vi "Simple Event Driven Example.vi"() -> ()   [LabVIEW 2013]
uses:
  lightfield-automation-labview/LightField Automation.lvclass
panel:
  in  "Load":bool
  in  "Experiment Name":string
  in  "Preview":bool
  in  "Acquire":bool
  in  "Exposure Time (s)":dbl format="%_3p"
  out "Intensity Graph":dbl[][](graph)
  in  "Close Program":bool
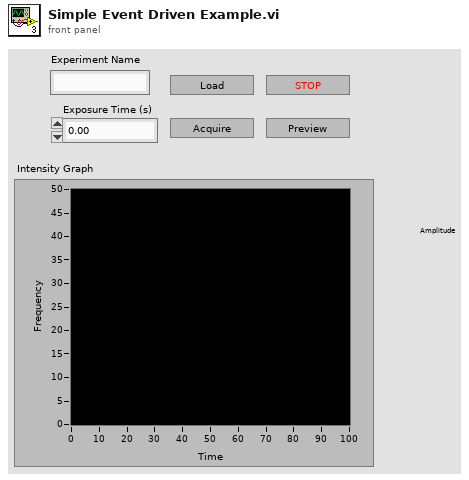
[diagram p1: front panel]
types:
  T1 = cluster{"Image":dbl[][][], "Frame Size":cluster{"F":i32, "Y":i32, "X":i32}}[]
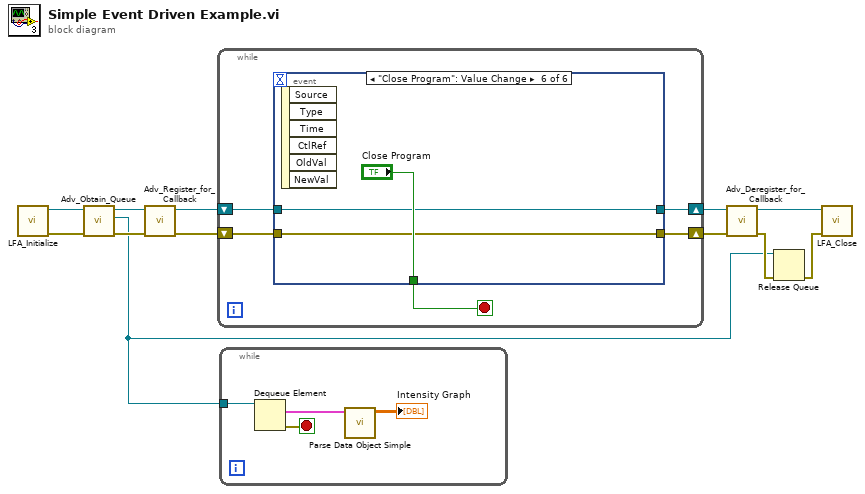
[diagram p0: block diagram]
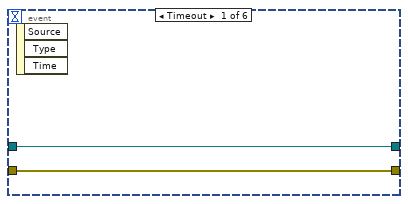
[diagram p2: hidden frame]
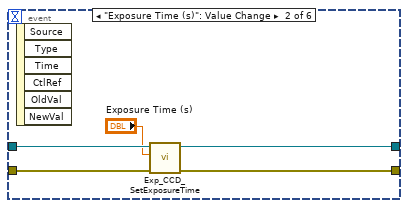
[diagram p3: hidden frame]
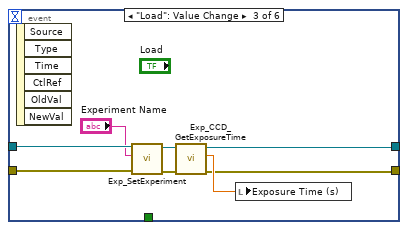
[diagram p4: hidden frame]
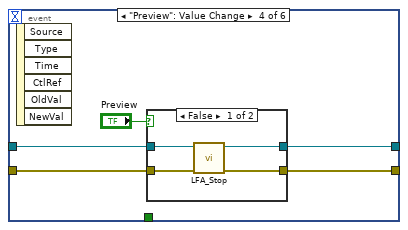
[diagram p5: hidden frame]
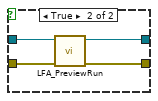
[diagram p6: hidden frame]
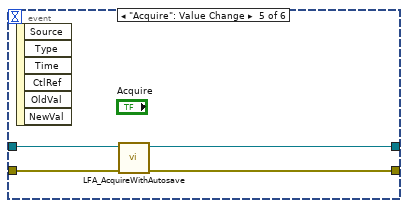
[diagram p7: hidden frame]
diagram:
  n1 = call "LFA_Initialize.vi"() -> ("error out"=w11:errorcluster, "LightField Automation out"=w12:refnum<class "LightField Automation.lvclass">)  [unwired: 10 in]
  n2 = call "Adv_Obtain_Queue.vi"("error in (no error)"=w11, "LightField Automation in"=w12) -> ("error out"=w9:errorcluster, "Queue Reference"=w1:refnum<queue>, "LightField Automation out"=w10:refnum<class "LightField Automation.lvclass">)  [unwired: 7 in]
  n3 = call "Adv_Register_for_Callback.vi"("error in (no error)"=w9, "LightField Automation in"=w10) -> ("error out"=w8:errorcluster, "LightField Automation out"=w7:refnum<class "LightField Automation.lvclass">)  [unwired: 8 in]
  n4 = while {
    shift-right: [w14] -> w6
    shift-left: w8 -> [w13]
    shift-right: [w15] -> w5
    shift-left: w7 -> [w16]
    stop <- w17 stop-if-true
    n5 = event shown="[5] \"Close Program\": Value Change" {
      selector: _ -> [_ _ _ _ _ _]
      dyn-events: _ -> [_ _ _ _ _ _]
      timeout: _ -> [_ _ _ _ _ _]
      tunnel: [_ _ _ _ _ "Close Program"] -> w17
      tunnel: w16 -> [w19 w24 w32 w34 w49 w51]
      tunnel: [w19 w21 w25 w35 w47 w51] -> w15
      tunnel: [w18 w22 w26 w36 w46 w50] -> w14
      tunnel: w13 -> [w18 w23 w31 w33 w48 w50]
      event Timeout {
        n6 = event-data() -> ()  [unwired: 1 in, 3 out]
      }
      event "Exposure Time (s)": Value Change {
        n7 = event-data() -> ()  [unwired: 1 in, 6 out]
        n8 = call "Exp_CCD_SetExposureTime.vi"("error in (no error)"=w23, "Exposure Time (s)"="Exposure Time (s)", "LightField Automation in"=w24) -> ("error out"=w22:errorcluster, "LightField Automation out"=w21:refnum<class "LightField Automation.lvclass">)  [unwired: 7 in]
      }
      event "Load": Value Change {
        n9 = event-data() -> ()  [unwired: 1 in, 6 out]
        n10 = call "Exp_SetExperiment.vi"("error in (no error)"=w31, "ExperimentName"="Experiment Name", "LightField Automation in"=w32) -> ("error out"=w29:errorcluster, "LightField Automation out"=w28:refnum<class "LightField Automation.lvclass">)  [unwired: 7 in]
        n11 = call "Exp_CCD_GetExposureTime.vi"("error in (no error)"=w29, "LightField Automation in"=w28) -> ("error out"=w26:errorcluster, "Exposure Time (s)"=w27:dbl, "LightField Automation out"=w25:refnum<class "LightField Automation.lvclass">)  [unwired: 7 in]
        n12 = local write "Exposure Time (s)"(w27) -> ()
      }
      event "Preview": Value Change {
        n13 = event-data() -> ()  [unwired: 1 in, 6 out]
        n14 = case shown="False" "Preview" {
          tunnel: [w38 w45] -> w36
          tunnel: [w39 w44] -> w35
          tunnel: w34 -> [w41 w43]
          tunnel: w33 -> [w40 w42]
          frame False {
            n15 = call "LFA_Stop.vi"("error in (no error)"=w40, "LightField Automation in"=w41) -> ("error out"=w38:errorcluster, "LightField Automation out"=w39:refnum<class "LightField Automation.lvclass">)  [unwired: 8 in]
          }
          frame True {
            n16 = call "LFA_PreviewRun.vi"("error in (no error)"=w42, "LightField Automation in"=w43) -> ("error out"=w45:errorcluster, "LightField Automation out"=w44:refnum<class "LightField Automation.lvclass">)  [unwired: 8 in]
          }
        }
      }
      event "Acquire": Value Change {
        n17 = event-data() -> ()  [unwired: 1 in, 6 out]
        n18 = call "LFA_AcquireWithAutosave.vi"("error in (no error)"=w48, "LightField Automation in"=w49) -> ("error out"=w46:errorcluster, "LightField Automation out"=w47:refnum<class "LightField Automation.lvclass">)  [unwired: 7 in, 1 out]
      }
      event "Close Program": Value Change {
        n19 = event-data() -> ()  [unwired: 1 in, 6 out]
      }
    }
  }
  n20 = while {
    tunnel: w1 -> [w56]
    stop <- w55 stop-if-true
    n21 = Dequeue Element(queue=w56) -> (element=w54:T1, error out=w55:errorcluster)  [unwired: 2 in, 2 out]
    n22 = call "Parse Data Object Simple.vi"("Data"=w54) -> ("ROI 1, Frame 1"=→"Intensity Graph":dbl[][])  [unwired: 9 in, 1 out]
  }
  n23 = call "Adv_Deregister_for_Callback.vi"("error in (no error)"=w6, "LightField Automation in"=w5) -> ("error out"=w4:errorcluster, "LightField Automation out"=w2:refnum<class "LightField Automation.lvclass">)  [unwired: 8 in]
  n24 = Release Queue(queue=w1, error in (no error)=w4) -> (error out=w3:errorcluster)  [unwired: 1 in, 2 out]
  n25 = call "LFA_Close.vi"("error in (no error)"=w3, "LightField Automation in"=w2) -> ()  [unwired: 8 in, 2 out]
